vi "Module Cleanup.vi"(8 "error in (no error)":errorcluster, 11 "Historian Module in":refnum<class "Historian Module.lvclass">) -> (0 "error out":errorcluster, 3 "Historian Module out":refnum<class "Historian Module.lvclass">)   [LabVIEW 2020, in "VolatusHistorian.lvlib" / "Historian Module.lvclass"]
uses:
  Historian Module.lvclass
  Historian Module.lvclass/Historian Module.ctl
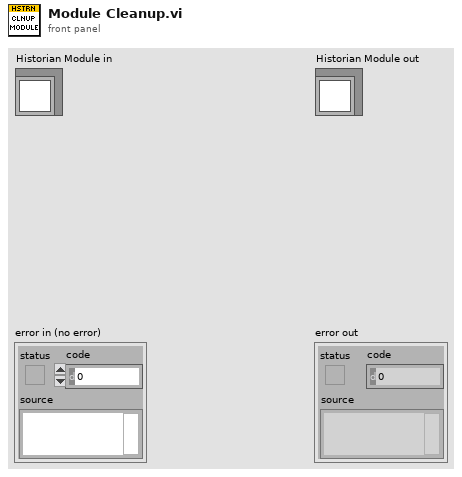
[diagram p1: front panel]
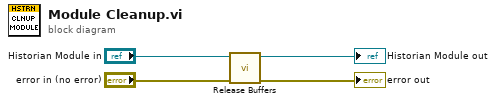
[diagram p0: block diagram]
diagram:
  n1 = call "Release Buffers.vi"("error in (no error)"="error in (no error)", "Historian Module in"="Historian Module in") -> ("error out"=→"error out":errorcluster, "Historian Module out"=→"Historian Module out":refnum<class "Historian Module.lvclass">)  [unwired: 8 in]
